vi "Find Fiducials.vi"(7 "Image Prefix":string, 8 "error in (no error)":errorcluster, 10 "Fiducial Type":string, 11 "Gantry in":refnum<class "Gantry.lvclass">) -> (0 "error out":errorcluster, 1 "Fiducial Physical Positions":refnum<class "Vec3d.lvclass">[](array[class]), 2 "Fiducial Image Positions":refnum<class "Vec3d.lvclass">[](array[class]), 3 "Gantry out":refnum<class "Gantry.lvclass">, 4 "log out":string, 5 "Fiducial Image":T1)   [LabVIEW 2022 SP3, in "Gantry.lvclass"]
uses:
  Gantry.lvclass
  Vec3d Class/Vec3d.lvclass
  Utils/Type Definitions/Physical Image.ctl
  <vilib>/vision/Image Controls.llb/IMAQ Image.ctl
  FlexWorktable/FlexWorktable.lvclass
  Gantry.lvclass/Gantry.ctl
  Vision/Vision.lvlib
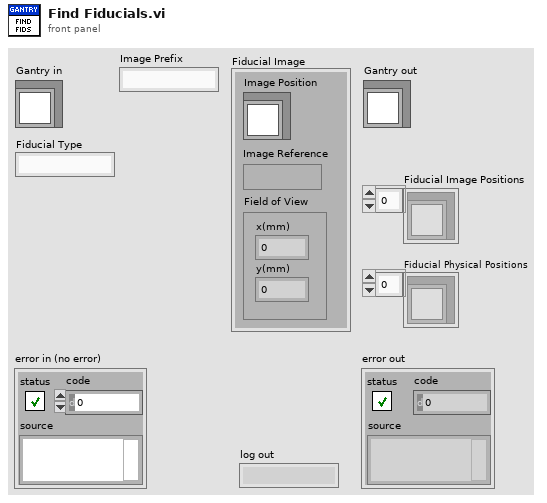
[diagram p1: front panel]
types:
  T1 = typedef "Physical Image.ctl" = cluster{"Image Position":refnum<class "Vec3d.lvclass">, "Image Reference":T2, "Field of View":cluster{"x(mm)":dbl, "y(mm)":dbl}}
  T2 = typedef "IMAQ Image.ctl" = refnum<image>
  T3 = typedef "FlexWorktable.lvclass/Camera State.ctl" = cluster{"Group":i32, "Open?":bool, "Driver":T4, "serial number":string, "Field of View":cluster{"x-mm":dbl, "y-mm":dbl}, "Rotation":T5, "Vertical Mirror":bool}
  T4 = typedef "Vision.lvlib/camera driver.ctl" = enum16{"none", "ueye", "wmf"}
  T5 = typedef "Camera Rotation.ctl" = enum16{"0", "90", "180", "270"}
  T6 = cluster{"x":dbl, "y":dbl, "image-x":dbl, "image-y":dbl}[]
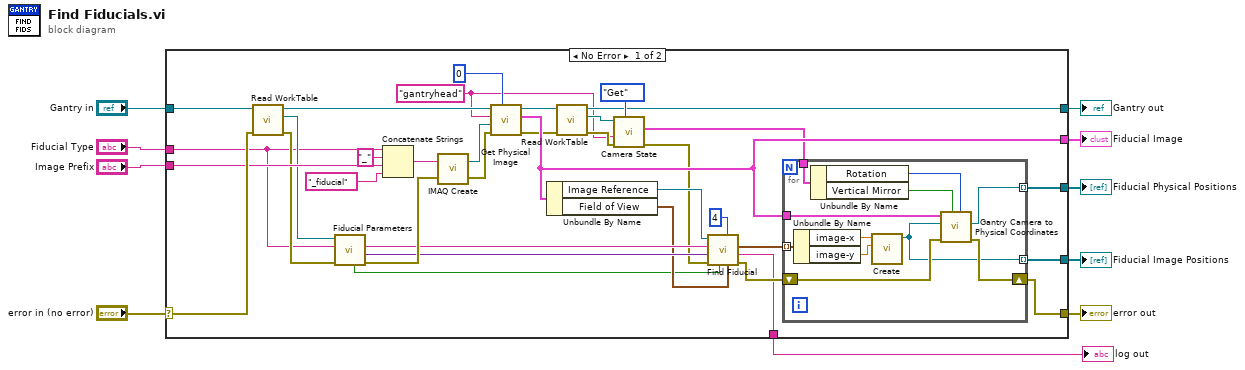
[diagram p0: block diagram]
diagram:
  n1 = case shown="No Error" "error in (no error)" {
    selector: "error in (no error)" -> [w42 w59]
    tunnel: [w13 w59] -> w9
    tunnel: [w18 w58] -> w7
    tunnel: "Gantry in" -> [w43 w58]
    tunnel: "Fiducial Type" -> [w38 _]
    tunnel: "Image Prefix" -> [w41 _]
    tunnel: [w25 _] -> w4
    tunnel: [w23 _] -> w3
    tunnel: [w24 _] -> w2
    tunnel: [w11 _] -> w1
    frame No Error {
      w12 = "gantryhead" ("Camera Name")
      n2 = call-dynamic "Read WorkTable.vi"("error in"=w42, "Gantry Class in"=w43) -> ("error out"=w39:errorcluster, "Worktable"=w40:refnum<class "FlexWorktable.lvclass">, "Gantry Class out"=w37:refnum<class "Gantry.lvclass">)  [unwired: 7 in]
      n3 = call-dynamic "Fiducial Parameters.vi"("error in (no error)"=w39, "Fiducial Type"=w38, "FlexWorktable in"=w40) -> ("error out"=w36:errorcluster, "Fiducial Parameters"=w32:variant, "Fiducial Method"=w33:string, "debug enable"=w30:bool)  [unwired: 4 in, 1 out]
      n4 = Concatenate Strings(w38, "_" ("string"), w41, "_fiducial" ("string")) -> (w46:string)
      n5 = call "IMAQ Create"("Image Name"=w46, "error in (no error)"=w36) -> ("New Image"=w35:T2, "error out"=w27:errorcluster)  [unwired: 3 in]
      n6 = call-dynamic "Get Physical Image.vi"("Delay(milliseconds)"=0, "error in"=w27, "Image In"=w35, "Camera Name"=w12, "Gantry in"=w37) -> ("error out"=w17:errorcluster, "Physical Image"=w23:T1, "Gantry out"=w19:refnum<class "Gantry.lvclass">)  [unwired: 4 in]
      n7 = Unbundle By Name(w23) -> ("Image Reference"=w29:T2, "Field of View"=w31:cluster{"x(mm)":dbl, "y(mm)":dbl})
      n8 = call-dynamic "Read WorkTable.vi"("error in"=w17, "Gantry Class in"=w19) -> ("error out"=w20:errorcluster, "Worktable"=w22:refnum<class "FlexWorktable.lvclass">, "Gantry Class out"=w18:refnum<class "Gantry.lvclass">)  [unwired: 7 in]
      n9 = call-dynamic "Camera State.vi"("Get/Set"=enum16{"Get", "Set"}."Get", "error in (no error)"=w20, "Camera Name"=w12, "FlexWorktable in"=w22) -> ("error out"=w16:errorcluster, "State"=w15:T3)  [unwired: 5 in, 1 out]
      n10 = call "Find Fiducial.vi"("Field of View"=w31, "Shrink Factor"=4, "debug"=w30, "error in"=w16, "Method Parameters"=w32, "Method Name"=w33, "Image"=w29) -> ("error out"=w14:errorcluster, "log out"=w11:string, "Fiducials"=w26:T6)  [unwired: 2 in]
      n11 = for {
        tunnel: w26 -> [w53] mode=indexing
        tunnel: [w47] -> w25 mode=indexing
        tunnel: [w48] -> w24 mode=indexing
        tunnel: w23 -> [w57]
        tunnel: w15 -> [w56]
        shift-right: [w49] -> w13
        shift-left: w14 -> [w50]
        n12 = Unbundle By Name(w53) -> ("image-x"=w52:dbl, "image-y"=w51:dbl)
        n13 = Unbundle By Name(w56) -> ("Rotation"=w54:T5, "Vertical Mirror"=w55:bool)
        n14 = call "Create.vi"("Y"=w51, "X"=w52) -> ("Vec3d Class out"=w47:refnum<class "Vec3d.lvclass">)  [unwired: 8 in, 1 out]
        n15 = call "Gantry Camera to Physical Coordinates.vi"("Rotation"=w54, "Vertical Mirror"=w55, "error in"=w50, "Image Coordinate"=w47, "Physical Image"=w57) -> ("error out"=w49:errorcluster, "Global Coordinate"=w48:refnum<class "Vec3d.lvclass">)  [unwired: 4 in, 1 out]
      }
    }
    frame Error {
    }
  }
  "error out" <- w9
  "Gantry out" <- w7
  "Fiducial Image Positions" <- w4
  "Fiducial Image" <- w3
  "Fiducial Physical Positions" <- w2
  "log out" <- w1
